vi "Draw Expanded IO.vi"(9 "State":T1, 11 "Picture In":picture) -> (3 "Picture":picture)   [LabVIEW 2020, in "Parallel Diagram Block.xnode"]
uses:
  Parallel Diagram Block.xnode
  Parallel Block/Parallel Block.lvlib
  Parallel Block/Terminal Mode.ctl
  Parallel Block/Value Mode.ctl
  Parallel Block/Value Type.ctl
  Parallel Block/Type Descriptor.ctl
  <vilib>/picture/picture.llb/imagedata.ctl
  Parallel Block/Direction.ctl
  State.ctl
  Parallel Block/Terminal Type.ctl
  Parallel Block/Type Mode.ctl
  Parallel Block/Manager Node.ctl
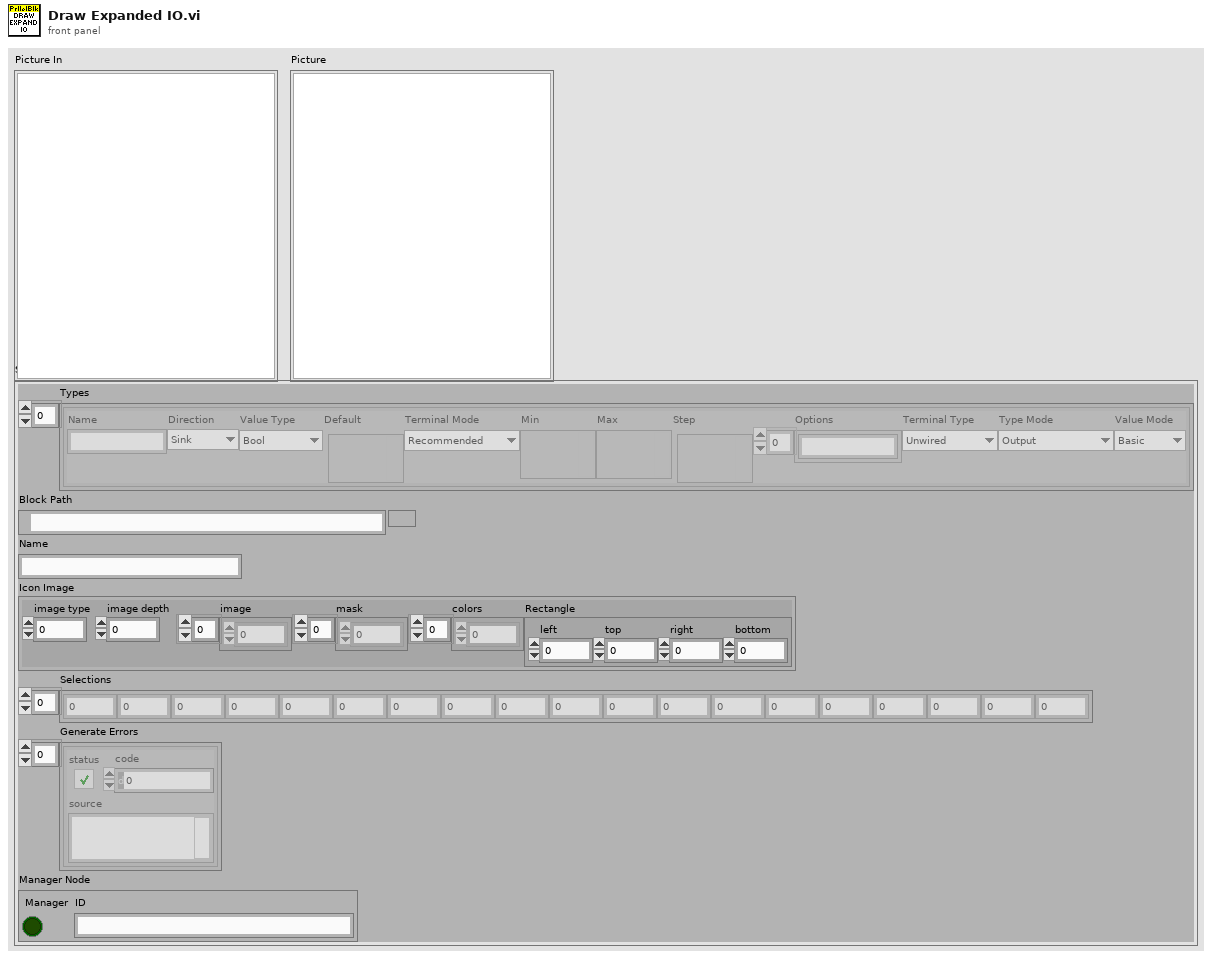
[diagram p1: front panel]
types:
  T1 = typedef "Parallel Diagram Block.xnode/State.ctl" = cluster{"Types":T2[], "Block Path":path, "Name":string, "Icon Image":T9, "Selections":i32[], "Generate Errors":errorcluster[], "Manager Node":T10}
  T2 = typedef "Parallel Block.lvlib/Type Descriptor.ctl" = cluster{"Name":string, "Direction":T3, "Value Type":T4, "Default":variant, "Terminal Mode":T5, "Min":variant, "Max":variant, "Step":variant, "Options":string[], "Terminal Type":T6, "Type Mode":T7, "Value Mode":T8}
  T3 = typedef "Parallel Block.lvlib/Direction.ctl" = enum16{"Sink", "Source"}
  T4 = typedef "Parallel Block.lvlib/Value Type.ctl" = enum16{"Unknown", "Bool", "U8", "U16", "U32", "U64", "I8", "I16", "I32", "I64", "SGL", "DBL", "CSG", "CDB", "CDBWfm", "String", "DBLWfm"}
  T5 = typedef "Parallel Block.lvlib/Terminal Mode.ctl" = enum16{"Recommended", "Required", "None"}
  T6 = typedef "Parallel Block.lvlib/Terminal Type.ctl" = enum16{"Unwired", "BadType", "Connection", "Value", "Control Ref", "BadRefType"}
  T7 = typedef "Parallel Block.lvlib/Type Mode.ctl" = enum16{"Output", "Single - Strict", "Single - Coerced", "Stream"}
  T8 = typedef "Parallel Block.lvlib/Value Mode.ctl" = enum16{"Basic", "Range", "Select"}
  T9 = typedef "imagedata.ctl" = cluster{"image type":i32, "image depth":i32, "image":u8[], "mask":u8[], "colors":u32[], "Rectangle":cluster{"left":i16, "top":i16, "right":i16, "bottom":i16}}
  T10 = typedef "Parallel Block.lvlib/Manager Node.ctl" = cluster{"Manager":bool, "ID":string}
  T11 = cluster{"left":i16, "top":i16, "right":i16, "bottom":i16}
  T12 = cluster{"horizontal":enum16{"left", "center", "right"}, "vertical":enum16{"top", "center", "bottom"}}
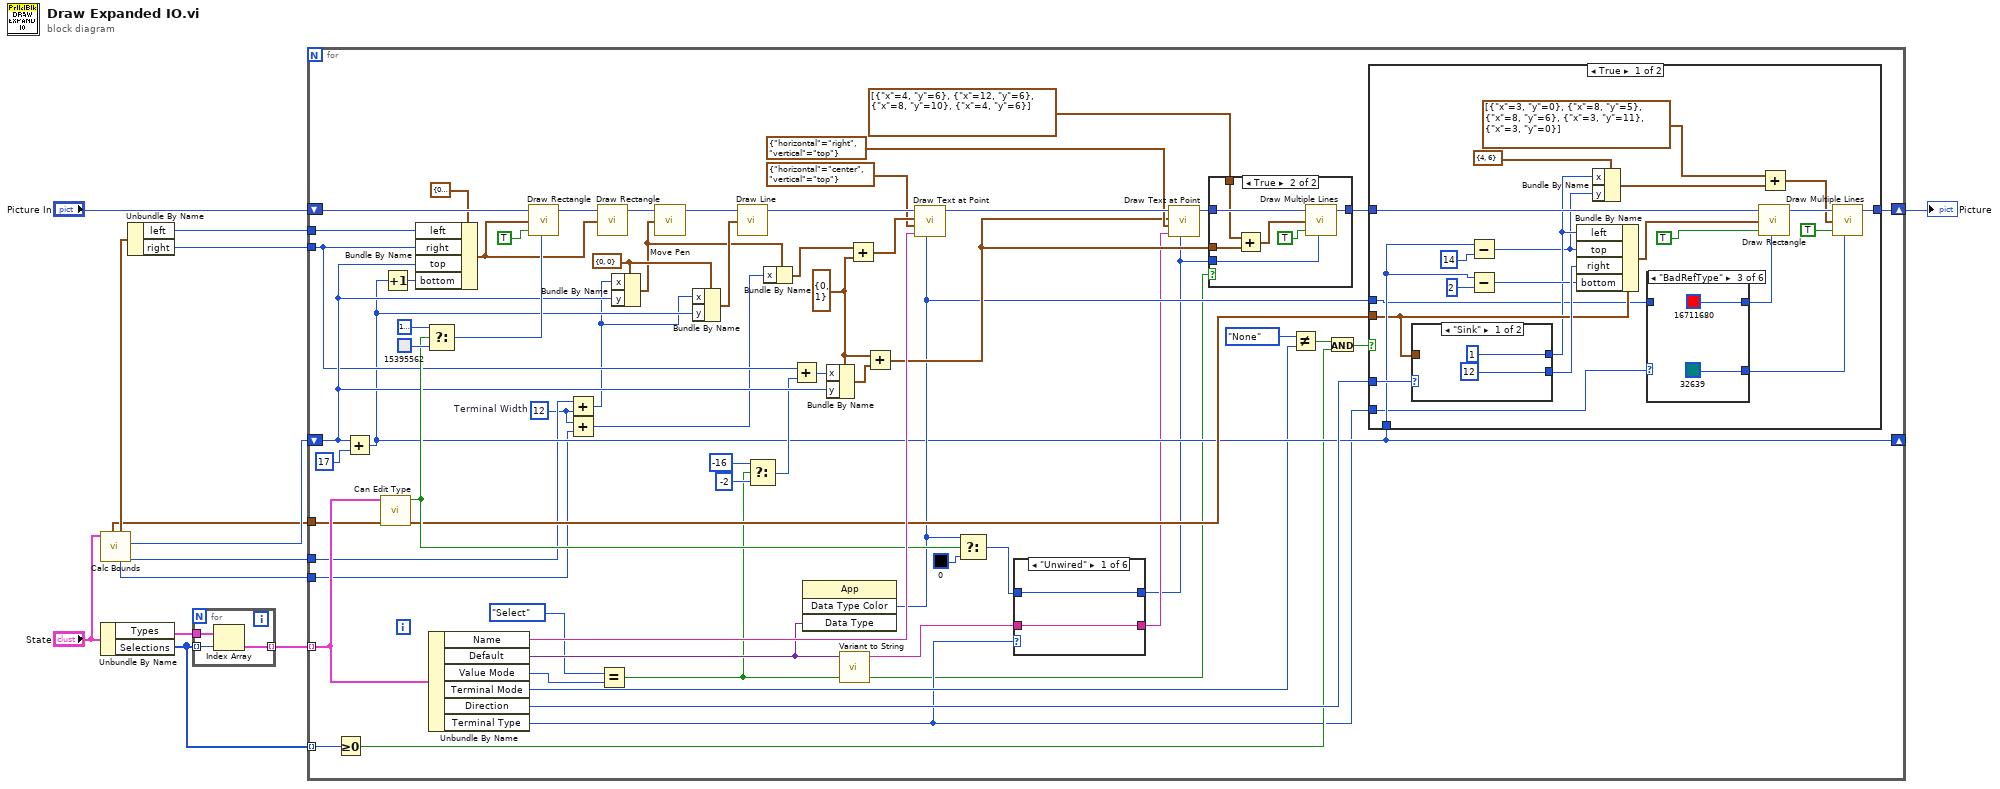
[diagram p0: block diagram]
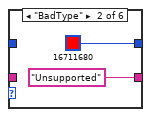
[diagram p2: hidden frame]
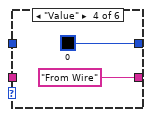
[diagram p4: hidden frame]
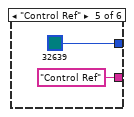
[diagram p5: hidden frame]
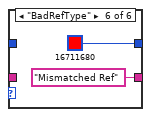
[diagram p6: hidden frame]
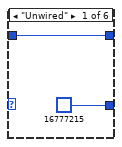
[diagram p7: hidden frame]
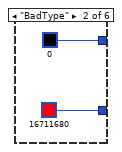
[diagram p8: hidden frame]
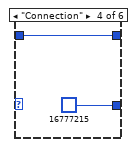
[diagram p9: hidden frame]
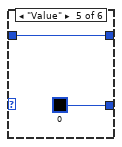
[diagram p10: hidden frame]
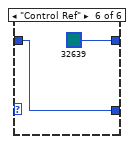
[diagram p11: hidden frame]
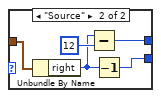
[diagram p12: hidden frame]
diagram:
  n1 = call "Calc Bounds.vi"("State"="State") -> ("Name Width"=w2:i16, "Header"=w9:i32, "Name Center"=w1:i16, "Bounds Without Terminals"=w8:T11, "Full Bounds"=w4:T11)  [unwired: 4 in, 2 out]
  n2 = Unbundle By Name("State") -> ("Types"=w12:T2[], "Selections"=w3:i32[])
  n3 = Unbundle By Name(w8) -> ("left"=w6:i16, "right"=w7:i16)
  n4 = for {
    tunnel: w12 -> [w16]
    tunnel: w3 -> [w15] mode=indexing
    tunnel: [w14] -> w11 mode=indexing
    n5 = Index Array(array=w16, index=w15) -> (element=w14:T2)
  }
  n6 = for {
    tunnel: w11 -> [w64] mode=indexing
    shift-right: [w42] -> w5
    shift-left: "Picture In" -> [w78]
    shift-right: [w38] -> _
    shift-left: w9 -> [w54]
    tunnel: w6 -> [w76]
    tunnel: w7 -> [w53]
    tunnel: w4 -> [w41]
    tunnel: w3 -> [w33] mode=indexing
    tunnel: w2 -> [w25]
    tunnel: w1 -> [w22]
    w19 = i16 12  # Terminal Width
    w55 = cluster{"x":i16, "y":i16} {"x"=0, "y"=1} ("new position")
    w69 = cluster{"x":i16, "y":i16} {"x"=0, "y"=0} ("new position")
    n7 = Greater Or Equal To 0?(x=w33) -> (x >= 0?=w32:bool)
    n8 = Add(x=w54, y=17) -> (x+y=w38:i32)
    n9 = call "Can Edit Type.vi"("Type Descriptor"=w64) -> ("Can Edit?"=w58:bool)  [unwired: 10 in]
    n10 = Increment(x=w38) -> (x+1=w65:i32)
    n11 = Bundle By Name(cluster=T11 {"left"=0, "top"=0, "right"=0, "bottom"=0} ("rect"), "left"=w76, "right"=w53, "top"=w54, "bottom"=w65) -> (w71:T11)
    n12 = Select(t=u32 16777225 ("color(black)"), s=w58, f=u32 15395562 ("color(black)")) -> (s? t:f=w73:u32)
    n13 = Unbundle By Name(w64) -> ("Name"=w62:string, "Default"=w59:variant, "Value Mode"=w46:T8, "Terminal Mode"=w37:T5, "Direction"=w40:T3, "Terminal Type"=w31:T6)
    n14 = call <vilib>:"Draw Rectangle.vi"("picture"=w78, "rect"=w71, "fill?(F)"=TRUE, "color(black)"=w73) -> ("new picture"=w72:picture)  [unwired: 5 in]
    n15 = Add(x=w25, y=w19) -> (x+y=w20:i16)
    n16 = Add(x=w19, y=w22) -> (x+y=w21:i16)
    n17 = call <vilib>:"Draw Rectangle.vi"("picture"=w72, "rect"=w71) -> ("new picture"=w70:picture)  [unwired: 7 in]
    n18 = Equal?(x=Value_Mode."Select", y=w46) -> (x = y?=w18:bool)
    n19 = Bundle By Name(cluster=w69, "x"=w20, "y"=w54) -> (w24:cluster{"x":i16, "y":i16})
    n20 = call <vilib>:"Move Pen.vi"("new position"=w24, "picture"=w70) -> ("new picture"=w67:picture)  [unwired: 3 in]
    n21 = Bundle By Name(cluster=w69, "x"=w20, "y"=w38) -> (w68:cluster{"x":i16, "y":i16})
    n22 = call <vilib>:"Draw Line.vi"("picture"=w67, "end point"=w68) -> ("new picture"=w63:picture)  [unwired: 7 in]
    n23 = Select(t=i16 -16 ("x"), s=w18, f=i16 -2) -> (s? t:f=w48:i16)
    n24 = Bundle By Name(cluster=w24, "x"=w21) -> (w23:cluster{"x":i16, "y":i16})
    n25 = Add(x=w53, y=w48) -> (x+y=w49:i16)
    n26 = invoke class="App" method="Data Type Color"("Data Type"=w59) -> ("Data Type Color"=w39:u32)  [unwired: 3 in, 3 out]
    n27 = Bundle By Name(cluster=w55, "x"=w49, "y"=w54) -> (w56:cluster{"x":i16, "y":i16})
    n28 = call "Variant to String.vi"("Value"=w59) -> ("String"=w30:string)  [unwired: 10 in]
    n29 = Add(x=w23, y=w55) -> (x+y=w61:cluster{"x":i16, "y":i16})
    n30 = Add(x=w55, y=w56) -> (x+y=w44:cluster{"x":i16, "y":i16})
    n31 = call <vilib>:"Draw Text at Point.vi"("text color(black)"=w39, "text"=w62, "alignment(left, top)"=T12 {"horizontal"=enum."center", "vertical"=enum."top"}, "origin"=w61, "picture"=w63) -> ("new picture"=w60:picture)  [unwired: 5 in, 1 out]
    n32 = Select(t=w39, s=w58, f=u32 0 ("color(black)")) -> (s? t:f=w28:u32)
    n33 = case shown="\"Unwired\"" w31 {
      tunnel: w30 -> [w81 _ w85 _ _ _]
      tunnel: [w81 "Unsupported" w85 "From Wire" ("String") "Control Ref" ("String") "Mismatched Ref" ("String")] -> w29
      tunnel: w28 -> [w80 _ w84 _ _ _]
      tunnel: [w80 u32 16711680 ("color(black)") w84 u32 0 ("color(black)") u32 32639 ("color(black)") u32 16711680 ("color(black)")] -> w27
      frame "Unwired" {
      }
      frame "BadType" {
      }
      frame "Connection" {
      }
      frame "Value" {
      }
      frame "Control Ref" {
      }
      frame "BadRefType" {
      }
    }
    n34 = call <vilib>:"Draw Text at Point.vi"("text color(black)"=w27, "text"=w29, "alignment(left, top)"=T12 {"horizontal"=enum."right", "vertical"=enum."top"}, "origin"=w44, "picture"=w60) -> ("new picture"=w47:picture)  [unwired: 5 in, 1 out]
    n35 = case shown="True" w18 {
      tunnel: w47 -> [w135 w142]
      tunnel: [w135 w141] -> w43
      tunnel: cluster{"x":i16, "y":i16}[] [{"x"=4, "y"=6}, {"x"=12, "y"=6}, {"x"=8, "y"=10}, {"x"=4, "y"=6}] ("line endpoints") -> [_ w138]
      tunnel: w44 -> [_ w139]
      tunnel: w27 -> [_ w136]
      frame False {
      }
      frame True {
        n36 = Add(x=w138, y=w139) -> (x+y=w137:cluster{"x":i16, "y":i16}[])
        n37 = call <vilib>:"Draw Multiple Lines.vi"("picture"=w142, "line endpoints"=w137, "fill?(F)"=TRUE, "color(black)"=w136) -> ("new picture"=w141:picture)  [unwired: 5 in]
      }
    }
    n38 = Not Equal?(x=Terminal_Mode."None", y=w37) -> (x != y?=w35:bool)
    n39 = And(x=w35, y=w32) -> (x .and. y?=w34:bool)
    n40 = case shown="True" w34 {
      tunnel: w43 -> [w114 w134]
      tunnel: [w102 w134] -> w42
      tunnel: w41 -> [w105 _]
      tunnel: w40 -> [w111 _]
      tunnel: w31 -> [w104 _]
      tunnel: w39 -> [w93 _]
      tunnel: w38 -> [w108 _]
      frame True {
        n41 = case shown="\"Sink\"" w111 {
          tunnel: [i16 1 ("y") w131] -> w99
          tunnel: [i16 12 ("y") w129] -> w110
          tunnel: w105 -> [_ w133]
          frame "Sink" {
          }
          frame "Source" {
            n42 = Unbundle By Name(w133) -> ("right"=w130:i16)
            n43 = Subtract(x=w130, y=i16 12) -> (x-y=w131:i16)
            n44 = Decrement(x=w130) -> (x-1=w129:i16)
          }
        }
        n45 = Subtract(x=w108, y=14) -> (x-y=w98:i32)
        n46 = Subtract(x=w108, y=2) -> (x-y=w107:i32)
        n47 = Bundle By Name(cluster=w105, "left"=w99, "top"=w98, "right"=w110, "bottom"=w107) -> (w106:T11)
        n48 = Bundle By Name(cluster=cluster{"x":i16, "y":i16} {"x"=4, "y"=6}, "x"=w99, "y"=w98) -> (w97:cluster{"x":i16, "y":i16})
        n49 = case shown="\"BadRefType\"" w104 {
          tunnel: [u32 16777215 ("color(black)") u32 16711680 ("color(black)") u32 32639 ("color(black)") u32 16777215 u32 0 ("color(black)") w125] -> w101
          tunnel: w93 -> [w115 _ _ w121 w124 w125]
          tunnel: [w115 u32 0 ("Data Type Color") u32 16711680 ("Data Type Color") w121 w124 u32 32639 ("color(black)")] -> w92
          frame "Unwired" {
          }
          frame "BadType" {
          }
          frame "BadRefType" {
          }
          frame "Connection" {
          }
          frame "Value" {
          }
          frame "Control Ref" {
          }
        }
        n50 = call <vilib>:"Draw Rectangle.vi"("picture"=w114, "rect"=w106, "fill?(F)"=TRUE, "color(black)"=w92) -> ("new picture"=w103:picture)  [unwired: 5 in]
        n51 = Add(x=cluster{"x":i16, "y":i16}[] [{"x"=3, "y"=0}, {"x"=8, "y"=5}, {"x"=8, "y"=6}, {"x"=3, "y"=11}, {"x"=3, "y"=0}] ("line endpoints"), y=w97) -> (x+y=w95:cluster{"x":i16, "y":i16}[])
        n52 = call <vilib>:"Draw Multiple Lines.vi"("picture"=w103, "line endpoints"=w95, "fill?(F)"=TRUE, "color(black)"=w101) -> ("new picture"=w102:picture)  [unwired: 5 in]
      }
      frame False {
      }
    }
  }
  "Picture" <- w5
